vi "Find BG Color Peak.vi"(11 "24-bit pixmap":u32[][](array[numeric]) format="%x") -> (3 "BG color value":u32)   [LabVIEW 2020, in "lv_icon.lvlib"]
doc: "Find the color that is supposely considered as the Background."
uses:
  lv_icon.lvlib
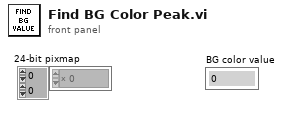
[diagram p1: front panel]
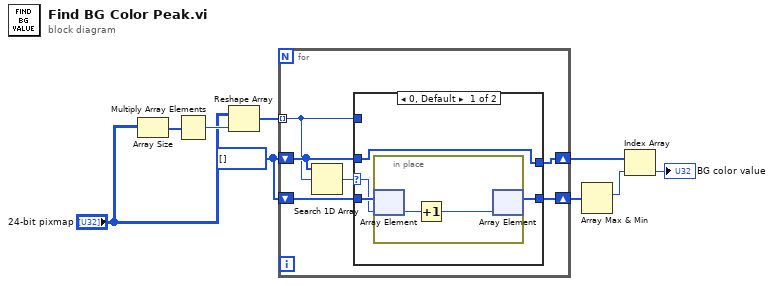
[diagram p0: block diagram]
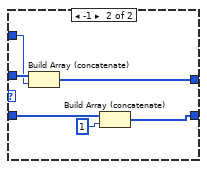
[diagram p2: hidden frame]
diagram:
  w6 = i32[] []
  n1 = Array Size(array="24-bit pixmap") -> (size(s)=w9:i32[])
  n2 = Multiply Array Elements(1:w9) -> (0:w8:i32)
  n3 = Reshape Array("24-bit pixmap", w8) -> (w7:u32[])
  n4 = for {
    tunnel: w7 -> [w12] mode=indexing
    shift-right: [w10] -> w5
    shift-left: w6 -> [w14]
    shift-right: [w11] -> w4
    shift-left: w6 -> [w13]
    n5 = Search 1D Array(1D array=w13, element=w12) -> (index of element=w15:i32)  [unwired: 1 in]
    n6 = case shown="0, Default" w15 {
      selector: w15 -> [w17 _]
      tunnel: w14 -> [w18 w24]
      tunnel: w13 -> [w19 w27]
      tunnel: w12 -> [_ w26]
      tunnel: [w19 w25] -> w11
      tunnel: [w16 w22] -> w10
      frame 0, Default {
        n7 = in-place {
          n8 = in-place-array #1(w18, w17) -> (w21:i32)
          n9 = Increment(x=w21) -> (x+1=w20:i32)
          n10 = in-place-array #1(w20) -> (w16:i32[])  [unwired: 1 out]
        }
      }
      frame -1 {
        n11 = Build Array (concatenate)(w27, w26) -> (w25:u32[])
        n12 = Build Array (concatenate)(w24, 1) -> (w22:i32[])
      }
    }
  }
  n13 = Array Max & Min(array=w5) -> (max index (indices)=w3:i32)  [unwired: 3 out]
  n14 = Index Array(array=w4, index=w3) -> (element=→"BG color value":u32)
